vi "ISET Read.vi"(8 "error in (no error)":errorcluster, 10 "Channel":T2, 11 "refnum in":T1) -> (0 "error out":errorcluster, 1 "Iset?":dbl, 2 "sIset":string, 3 "refnum out":T1, 4 "question out":string)   [LabVIEW 2020, in "Korad KA3305P.lvlib"]
uses:
  Korad KA3305P.lvlib
  Channels.ctl
  Reference.ctl
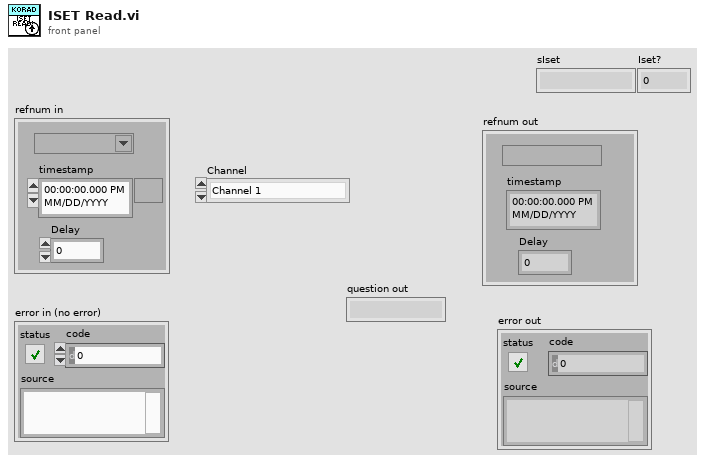
[diagram p1: front panel]
types:
  T1 = typedef "Korad KA3305P.lvlib/Reference.ctl" = cluster{"refnum":refnum<visa-resource-name>, "timestamp":timestamp, "Delay":dbl}
  T2 = typedef "Korad KA3305P.lvlib/Channels.ctl" = enum16{"Channel 1", "Channel 2"}
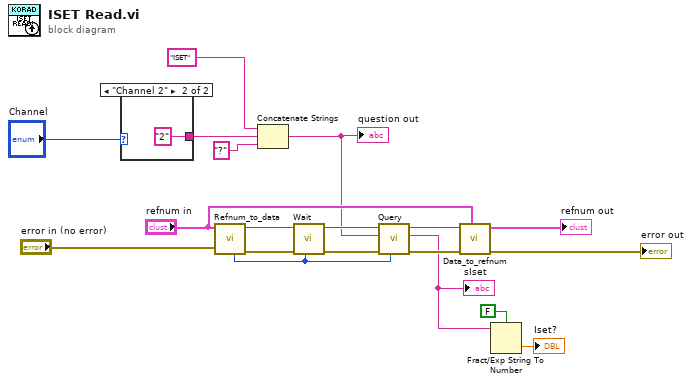
[diagram p0: block diagram]
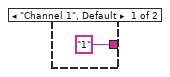
[diagram p2: hidden frame]
diagram:
  n1 = case shown="\"Channel 2\"" "Channel" {
    tunnel: ["1" "2"] -> w17
    frame "Channel 1", Default {
    }
    frame "Channel 2" {
    }
  }
  n2 = call "Refnum_to_data.vi"("error in (no error)"="error in (no error)", "refnum in"="refnum in") -> ("error out"=w14:errorcluster, "DAQ refnum out"=w13:refnum<visa-resource-name>, "delay out"=w4:u32)  [unwired: 7 in]
  n3 = Concatenate Strings("ISET" ("string"), w17, "?" ("string")) -> (w7:string)
  "question out" <- w7
  n4 = call "Wait.vi"("milliseconds to wait"=w4, "error in (no error)"=w14, "refnum in"=w13) -> ("error out"=w8:errorcluster, "refnum out"=w9:refnum<visa-resource-name>)  [unwired: 7 in]
  n5 = call "Query.vi"("delay (55ms)"=w4, "error in (no error)"=w8, "data in"=w7, "refnum in"=w9) -> ("error out"=w5:errorcluster, "data out"=w3:string, "refnum out"=w6:refnum<visa-resource-name>)  [unwired: 5 in]
  "sIset" <- w3
  n6 = call "Data_to_refnum.vi"("refnum in"="refnum in", "error in (no error)"=w5, "DAQ refnum in"=w6) -> ("error out"=→"error out":errorcluster, "refnum out"=→"refnum out":T1)  [unwired: 7 in]
  n7 = Fract/Exp String To Number(use system decimal point (T)=FALSE, string=w3) -> (number=→"Iset?":dbl)  [unwired: 2 in, 1 out]
